vi "Confirm Device Update.vi"(10 "Updated Device":refnum<class "Device.lvclass">, 11 "Existing Device":refnum<class "Device.lvclass">) -> (2 "Device":refnum<class "Device.lvclass">, 3 "Result":T1)   [LabVIEW 2020, in "PicoG-App.lvlib" / "DeviceListPanel.lvclass"]
uses:
  DeviceListPanel.lvclass
  Device/Device.lvclass
  Device Update Action.ctl
  DeviceListPanel.lvclass/DeviceListPanel.ctl
panel:
  in  "Cancel":bool
  in  "Goto Existing":bool
  in  "Update":bool
  out "New Alias":string
  out "Known Alias":string
  # "This device is already tracked by picoG.\n\nDo you want to update the existing entry?"
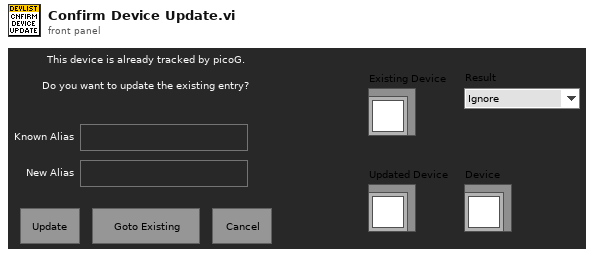
[diagram p1: front panel]
types:
  T1 = typedef "PicoG-App.lvlib/DeviceListPanel.lvclass/Device Update Action.ctl" = enum16{"Ignore", "Update", "Show Existing"}
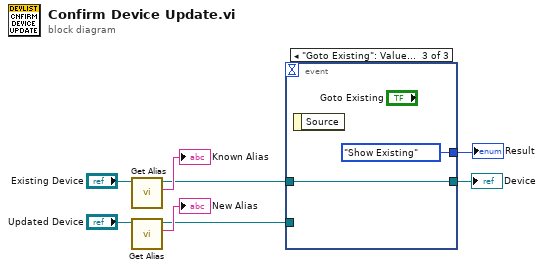
[diagram p0: block diagram]
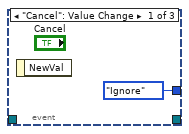
[diagram p2: hidden frame]
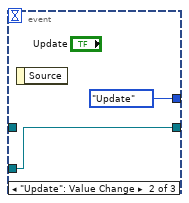
[diagram p3: hidden frame]
diagram:
  n1 = call "Get Alias.vi"("Device in"="Existing Device") -> ("Alias"=→"Known Alias":string, "Device out"=w2:refnum<class "Device.lvclass">)  [unwired: 8 in, 1 out]
  n2 = call "Get Alias.vi"("Device in"="Updated Device") -> ("Alias"=→"New Alias":string, "Device out"=w3:refnum<class "Device.lvclass">)  [unwired: 8 in, 1 out]
  n3 = event shown="[2] \"Goto Existing\": Value Change" {
    selector: _ -> [_ _ _]
    dyn-events: _ -> [_ _ _]
    timeout: _ -> [_ _ _]
    tunnel: [Device_Update_Action."Ignore" ("Result") Device_Update_Action."Update" ("Result") Device_Update_Action."Show Existing" ("Result")] -> w4
    tunnel: w3 -> [_ w10 _]
    tunnel: w2 -> [_ _ w12]
    tunnel: [_ w10 w12] -> w1
    event "Cancel": Value Change {
      n4 = event-data() -> ()  [unwired: 1 in, 1 out]
    }
    event "Update": Value Change {
      n5 = event-data() -> ()  [unwired: 1 in, 1 out]
    }
    event "Goto Existing": Value Change {
      n6 = event-data() -> ()  [unwired: 1 in, 1 out]
    }
  }
  "Device" <- w1
  "Result" <- w4
